vi "Get Resource Type.vi"(4 "SPI in":refnum<class "SPI.lvclass">) -> (7 "Resource Type":string)   [LabVIEW 2024, in "CTI.lvlib" / "SPI.lvclass"]
uses:
  SPI.lvclass
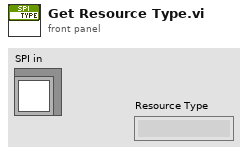
[diagram p1: front panel]
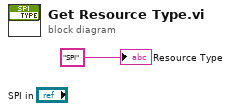
[diagram p0: block diagram]
diagram:
  "Resource Type" <- "SPI" ("Resource Type")
